vi "deadzoneCorrection.vi"(3 "u 2":dbl, 4 "u 1":dbl, 5 "u 0":dbl) -> (0 "out2":dbl, 1 "out1":dbl, 2 "out0":dbl)   [LabVIEW 2014]
uses:
  <vilib>/imath/engines/lvmath2/RunTimeEngine/NodeEndStatement/NIMS_NodeEndStatement_Output.vi
  <instcachedir>/0/NIMS_NodeEndStatement_Output_53EC0D466D134D7ABD903AC30B43404B.lvgen/NIMS_NodeEndStatement_Output_53EC0D466D134D7ABD903AC30B43404B_001.vi
  <vilib>/imath/engines/lvmath2/RunTimeEngine/ErrorHandling/NIMS_Finalize Error.vi
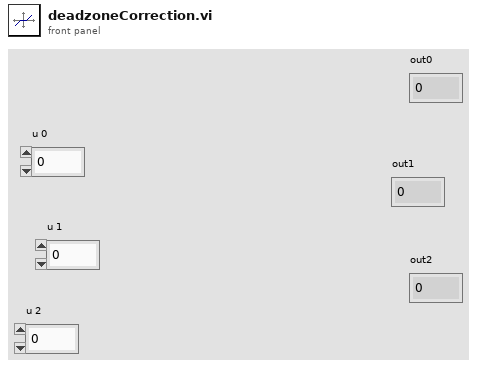
[diagram p1: front panel]
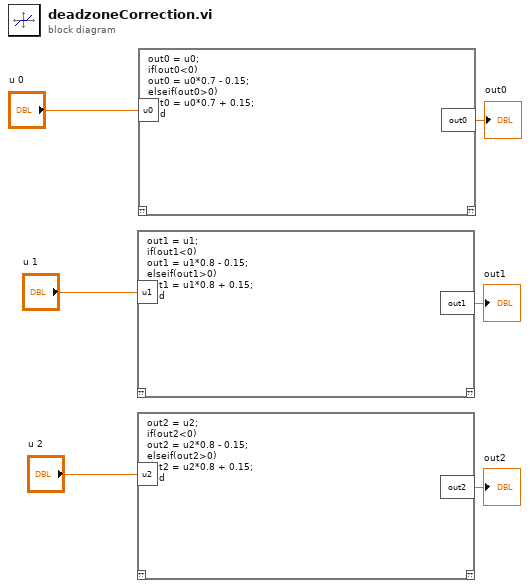
[diagram p0: block diagram]
diagram:
  n1 = mathscript code="out1 = u1;\nif(out1<0)\nout1 = u1*0.8 - 0.15;\nelseif(out1>0)\nout1 = u1*0.8 + 0.15;\nend"("u1"="u 1") -> ("out1"=→"out1":dbl)  [unwired: 1 in, 1 out]
  n2 = mathscript code="out2 = u2;\nif(out2<0)\nout2 = u2*0.8 - 0.15;\nelseif(out2>0)\nout2 = u2*0.8 + 0.15;\nend"("u2"="u 2") -> ("out2"=→"out2":dbl)  [unwired: 1 in, 1 out]
  n3 = mathscript code="out0 = u0;\nif(out0<0)\nout0 = u0*0.7 - 0.15;\nelseif(out0>0)\nout0 = u0*0.7 + 0.15;\nend"("u0"="u 0") -> ("out0"=→"out0":dbl)  [unwired: 1 in, 1 out]
